vi "__del__.vi"(8 "error in":errorcluster, 11 "Coarse Approach in":refnum<class "Coarse Approach.lvclass">) -> (0 "error out":errorcluster)   [LabVIEW 2020, in "Coarse Approach.lvclass"]
uses:
  Coarse Approach.lvclass
  Coarse Approach.lvclass/Coarse Approach.ctl
  Lock-In Amplifier/Lock-In Amplifier.lvclass
  Function Generator/Function Generator.lvclass
  Picomotor/Picomotor.lvclass
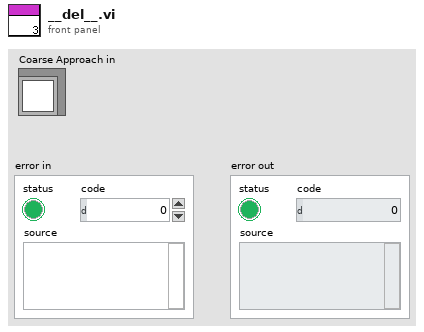
[diagram p1: front panel]
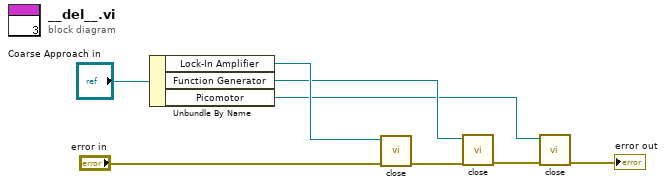
[diagram p0: block diagram]
diagram:
  n1 = Unbundle By Name("Coarse Approach in") -> ("Lock-In Amplifier"=w7:refnum<class "Lock-In Amplifier.lvclass">, "Function Generator"=w6:refnum<class "Function Generator.lvclass">, "Picomotor"=w3:refnum<class "Picomotor.lvclass">)
  n2 = call-dynamic "close.vi"("error in (no error)"="error in", "Instrument in"=w7) -> ("error out"=w4:errorcluster)  [unwired: 9 in]
  n3 = call-dynamic "close.vi"("error in (no error)"=w4, "Function Generator in"=w6) -> ("error out"=w2:errorcluster)  [unwired: 9 in]
  n4 = call-dynamic "close.vi"("error in (no error)"=w2, "Instrument in"=w3) -> ("error out"=→"error out":errorcluster)  [unwired: 9 in]
